vi "Dpc Pending Transactions.vi"(8 "error in (no error)":errorcluster, 9 "perc":i32, 10 "pctran":i32, 11 "hif":u32) -> (0 "error out":errorcluster, 1 "perc out":i32, 2 "pctran out":i32, 3 "hif out":u32, 5 "function return":i32)   [LabVIEW 2011, in "LVH-Adept.lvlib" / "DPCUTIL.lvlib"]
doc: "DPCAPI BOOL DpcPendingTransactions(HANDLE hif, INT32 * pctran, ERC * perc);"
uses:
  DPCUTIL.lvlib
  <vilib>/LabVIEW Hacker/Adept/Private/Resources/dpcutil.dll
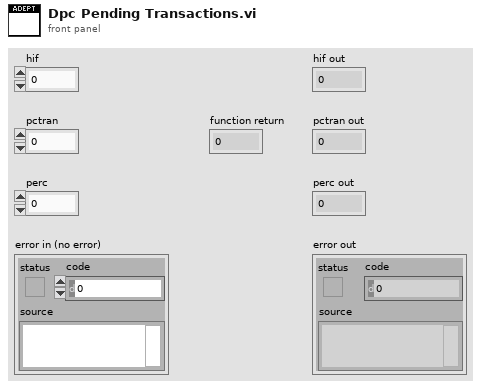
[diagram p1: front panel]
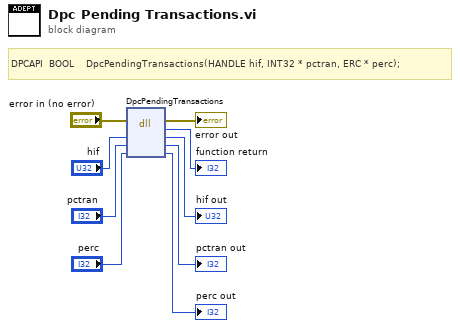
[diagram p0: block diagram]
diagram:
  # "DPCAPI  BOOL    DpcPendingTransactions(HANDLE hif, INT32 * pctran, ERC * perc);"
  n1 = dll-call lib="C:/Program Files (x86)/National Instruments/LabVIEW 2011/vi.lib/LabVIEW Hacker/Adept/Private/Resources/dpcutil.*" fn="DpcPendingTransactions"(error in="error in (no error)", "hif"="hif", "pctran"="pctran", "perc"="perc") -> (error out=→"error out":errorcluster, →"function return":i32, "hif"=→"hif out":u32, "pctran"=→"pctran out":i32, "perc"=→"perc out":i32)  [unwired: 2 in, 1 out]
